vi "CheckForSuccess.vi"(8 "error in":errorcluster, 11 "headers":string) -> (0 "error out":errorcluster, 3 "success":bool)   [LabVIEW 2017, in "LabVIEWHTTPClient.lvlib"]
uses:
  <vilib>/httpClient/LabVIEWHTTPClient.lvlib
  <vilib>/regexp/Match Regular Expression.xnode
panel:
  out "whole match":string
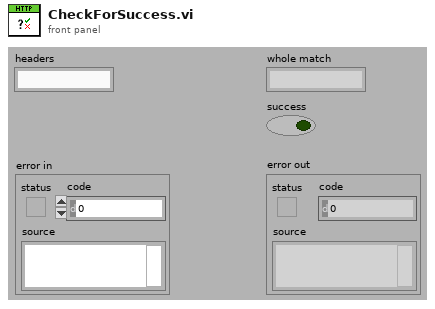
[diagram p1: front panel]
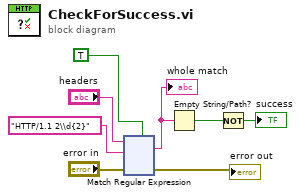
[diagram p0: block diagram]
diagram:
  n1 = xnode "Match Regular Expression"("input string"="headers", "regular expression"="HTTP/1.1 2\\d{2}", "error in"="error in", "multiline? (F)"=TRUE) -> ("whole match"=w5:string, "error out"=→"error out":errorcluster)  [unwired: 2 in, 3 out]
  "whole match" <- w5
  n2 = Empty String/Path?(string/path=w5) -> (empty?=w4:bool)
  n3 = Not(x=w4) -> (.not. x?=→"success":bool)
